vi "Area.vi"(8 "error in (no error)":errorcluster, 11 "Circle in":refnum<class "Circle.lvclass">) -> (0 "error out":errorcluster, 2 "rect":T1, 3 "Circle out":refnum<class "Circle.lvclass">)   [LabVIEW 2021, in "Picture2D.lvlib" / "Circle.lvclass"]
uses:
  Circle.lvclass
  Point/Point.lvclass
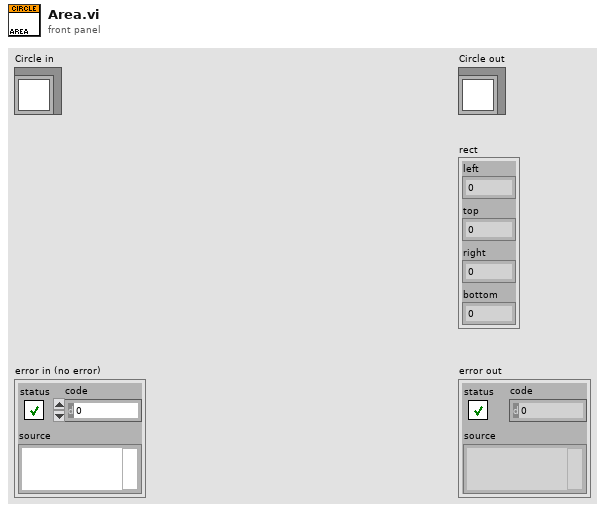
[diagram p1: front panel]
types:
  T1 = cluster{"left":i16, "top":i16, "right":i16, "bottom":i16}
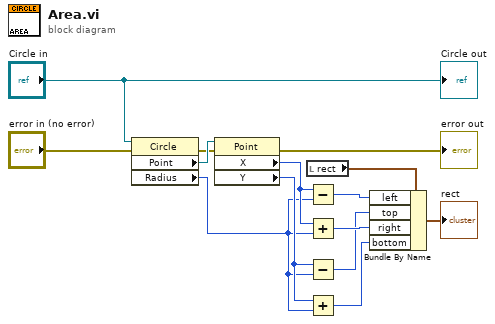
[diagram p0: block diagram]
diagram:
  n1 = property class="Circle"(reference="Circle in", error in="error in (no error)") -> (error out=w12:errorcluster, "Point"=w13:refnum<class "Point.lvclass">, "Radius"=w2:i16)  [unwired: 1 out]
  n2 = property class="Point"(reference=w13, error in=w12) -> (error out=→"error out":errorcluster, "X"=w6:i16, "Y"=w3:i16)  [unwired: 1 out]
  n3 = local read "rect"() -> (w8:T1)
  n4 = Subtract(x=w6, y=w2) -> (x-y=w7:i16)
  n5 = Add(x=w6, y=w2) -> (x+y=w5:i16)
  n6 = Subtract(x=w3, y=w2) -> (x-y=w4:i16)
  n7 = Add(x=w3, y=w2) -> (x+y=w1:i16)
  n8 = Bundle By Name(cluster=w8, "left"=w7, "top"=w4, "right"=w5, "bottom"=w1) -> (→"rect":T1)
  "Circle out" <- "Circle in"
